vi "Synth Set Amplitude.vi"(8 "error in (no error)":errorcluster, 9 "0 to 2.1 VRMS":dbl=2.1 min=0.0 max=2.5, 10 "DAQmx Device Name":tag="6251") -> (0 "error out":errorcluster)   [LabVIEW 2016]
uses:
  <vilib>/DAQmx/write.llb/DAQmx Write (Digital 1D Bool 1Chan 1Samp).vi
  <vilib>/DAQmx/create/channels.llb/DAQmx Create Channel (DO-Digital Output).vi
  <vilib>/DAQmx/miscellaneous.llb/DAQmx Fill In Error Info.vi
panel:
  out "size":i32
  out "Amp Word":u8[](array[numeric]) format="%08b"
  out "Amp int":i32
  out "Amp":u16 format="%016b"
  # "function          J7          P3\n              syn1 w clk       A0           3\n              syn1 D7           A1           5\n              syn2 w clk       A2           7\n              syn2 D7           A3           9\n              syn3 w clk       A4           4\n              syn3 D7           A5           6\n              syn1,2 FQ_UD  A6           8\n              syn3 FQ_UD     A7          10\n\n              Reset 1,2,3     B4          14\n\n              SCLK              B0           13\n              SYNC              B1           15\n              DIN                B2           17"
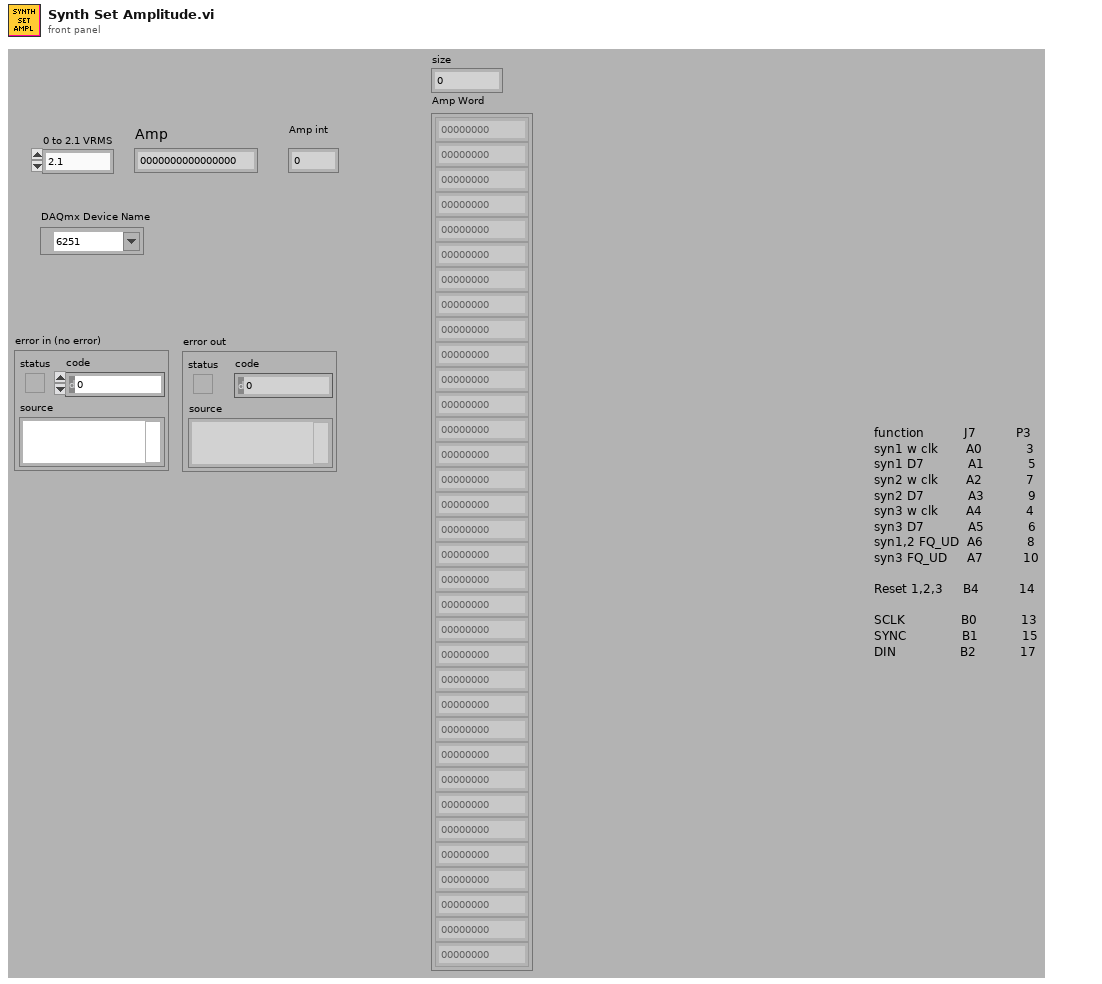
[diagram p1: front panel]
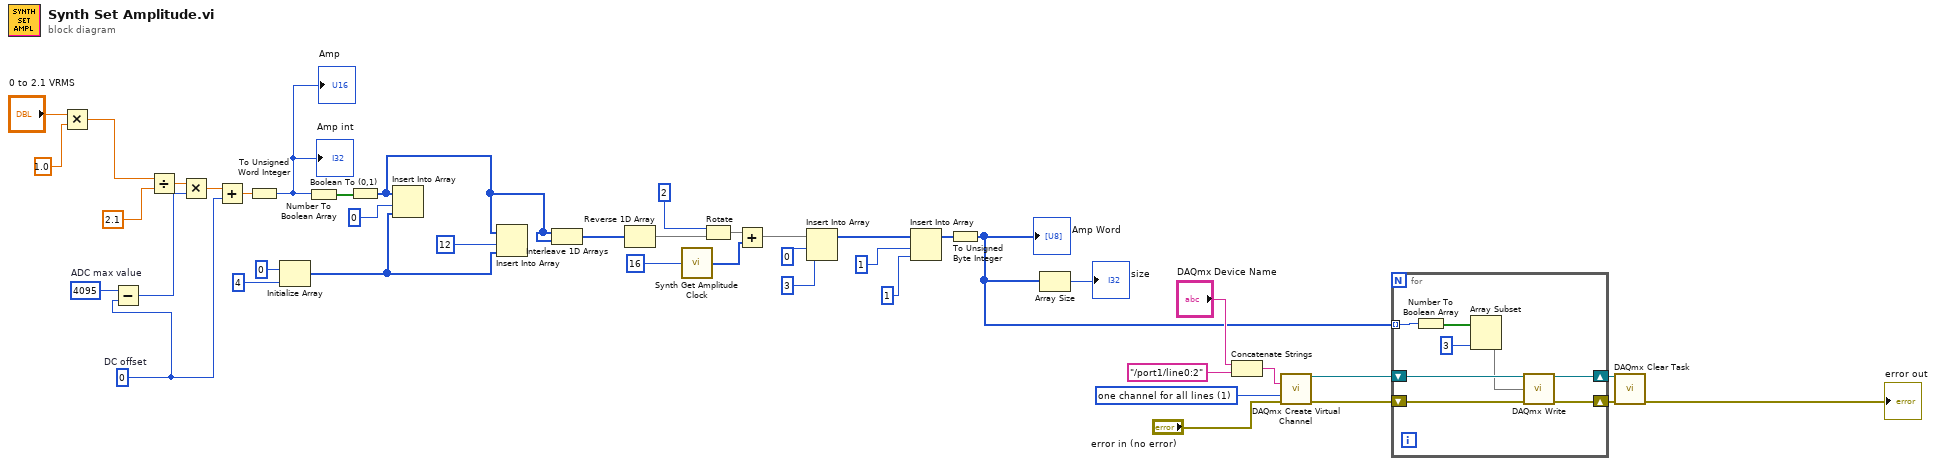
[diagram p0: block diagram]
diagram:
  w13 = 1 items=["one channel for each line", "one channel for all lines"] ("line grouping")
  w15 = i8 0  # DC offset
  w39 = u16 4095  # ADC max value
  n1 = Multiply(x="0 to 2.1 VRMS", y=1.0) -> (x*y=w4:dbl)
  n2 = Subtract(x=w39, y=w15) -> (x-y=w16:u16)
  n3 = Divide(x=w4, y=2.1) -> (x/y=w40:dbl)
  n4 = Multiply(x=w40, y=w16) -> (x*y=w18:dbl)
  n5 = Add(x=w18, y=w15) -> (x+y=w19:dbl)
  n6 = To Unsigned Word Integer(number=w19) -> (unsigned 16bit integer=w17:u16)
  "Amp" <- w17
  "Amp int" <- w17
  n7 = Initialize Array(u8 0 ("element"), 4 ("dimension size")) -> (w26:u8[])
  n8 = Number To Boolean Array(number=w17) -> (Boolean array=w43:bool[])
  n9 = Boolean To (0,1)(Boolean=w43) -> (0, 1=w5:i16[])
  n10 = Insert Into Array(array=w5, index=0, new element=w26) -> ()  [unwired: 1 out]
  n11 = Insert Into Array(array=w5, index=12, new element=w26) -> ()  [unwired: 1 out]
  n12 = Interleave 1D Arrays(w5, w5) -> (w22:i16[])
  n13 = Reverse 1D Array(array=w22) -> (reversed array=w21:i16[])
  n14 = call "Synth Get Amplitude Clock.vi"("Clk String Lngth"=16) -> ("TimingClock"=w27:u8[])
  n15 = Rotate(1:w21, 2:i8 2) -> (0:w23:i16[])
  n16 = Add(x=w23, y=w27) -> (x+y=w35:i16[])
  n17 = Insert Into Array(array=w35, index=0, new element=3 ("index")) -> (w31:i16[])
  n18 = Insert Into Array(array=w31, index=1, new element=1 ("index")) -> (w20:i16[])
  n19 = To Unsigned Byte Integer(number=w20) -> (unsigned 8bit integer=w1:u8[])
  "Amp Word" <- w1
  n20 = Array Size(array=w1) -> (size(s)=→"size":i32)
  n21 = Concatenate Strings("DAQmx Device Name", "/port1/line0:2") -> (w7:string)
  n22 = call-poly <vilib>:"DAQmx Create Virtual Channel.vi"("lines"=w7, "line grouping"=w13, "error in"="error in (no error)") -> ("task out"=w9:refnum<k21>, "error out"=w10:errorcluster)  [unwired: 2 in, 9 out]
  n23 = for {
    tunnel: w1 -> [w47] mode=indexing
    shift-right: [w50] -> w11
    shift-left: w9 -> [w48]
    shift-right: [w51] -> w12
    shift-left: w10 -> [w49]
    n24 = Number To Boolean Array(number=w47) -> (Boolean array=w45:bool[])
    n25 = Array Subset(array=w45, length=3) -> (w46:bool[])  [unwired: 1 in]
    n26 = call-poly <vilib>:"DAQmx Write.vi"("task/channels in"=w48, "data"=w46, "error in"=w49) -> ("task out"=w50:refnum<k21>, "error out"=w51:errorcluster)  [unwired: 10 in, 1 out]
  }
  n27 = call <vilib>:"DAQmx Clear Task.vi"("task in"=w11, "error in"=w12) -> ("error out"=→"error out":errorcluster)  [unwired: 13 out]
